vi "Controller Test Bench (9).vi"() -> ()   [LabVIEW 2022 SP3]
uses:
  <vilib>/sound2/lvsound2.llb/Sound Data Format.ctl
  <vilib>/Utility/error.llb/DialogType.ctl
  <vilib>/sound2/lvsound2.llb/Sampling Mode.ctl
  <vilib>/Analysis/4window.llb/windowTd.ctl
  <vilib>/DAQmx/read.llb/DAQmx Read (Analog 1D Wfm NChan NSamp).vi
  <vilib>/DAQmx/write.llb/DAQmx Write (Analog 1D DBL 1Chan NSamp).vi
  <vilib>/DAQmx/create/channels.llb/DAQmx Create Channel (AO-Voltage-Basic).vi
  <vilib>/DAQmx/create/channels.llb/DAQmx Create Channel (AI-Acceleration-Accelerometer).vi
  <vilib>/DAQmx/configure/timing.llb/DAQmx Timing (Sample Clock).vi
  <vilib>/DAQmx/miscellaneous.llb/DAQmx Fill In Error Info.vi
  <vilib>/DAQmx/configure/task.llb/DAQmx Configure Logging (TDMS).vi
  <vilib>/measure/maspectr.llb/FFT Spectrum (Mag-Phase) for N Chan.vi
  <vilib>/sound2/lvsound2.llb/Sound Output Set Volume (Single).vi
  <vilib>/sound2/lvsound2.llb/Sound Output Write (DBL Single).vi
  <vilib>/measure/NI_MAPro.lvlib
  <resource>/objmgr/daqmx.rc
  <vilib>/Analysis/NI_AALPro.lvlib
  <vilib>/measure/NI_MABase.lvlib
panel:
  in  "Gain":dbl
  in  "Setpoint":dbl
  out "Waveform Chart":waveform(dbl)[](graph)
  out "Numeric":i32
  in  "Output Noise":bool
  in  "reset signal":bool
  out "number of samples written per channel":u32
  in  "Active Control":bool
  in  "Log Data":bool
  out "Phase 2":cluster{"f0":dbl, "df":dbl, "phase":dbl[]}[](graph)
  out "Mag 2":cluster{"f0":dbl, "df":dbl, "magnitude":dbl[]}[](graph)
  in  "Show FFT":bool
  in  "Save FFT":bool
  in  "Start Acquisition":bool
  in  "Stop":bool
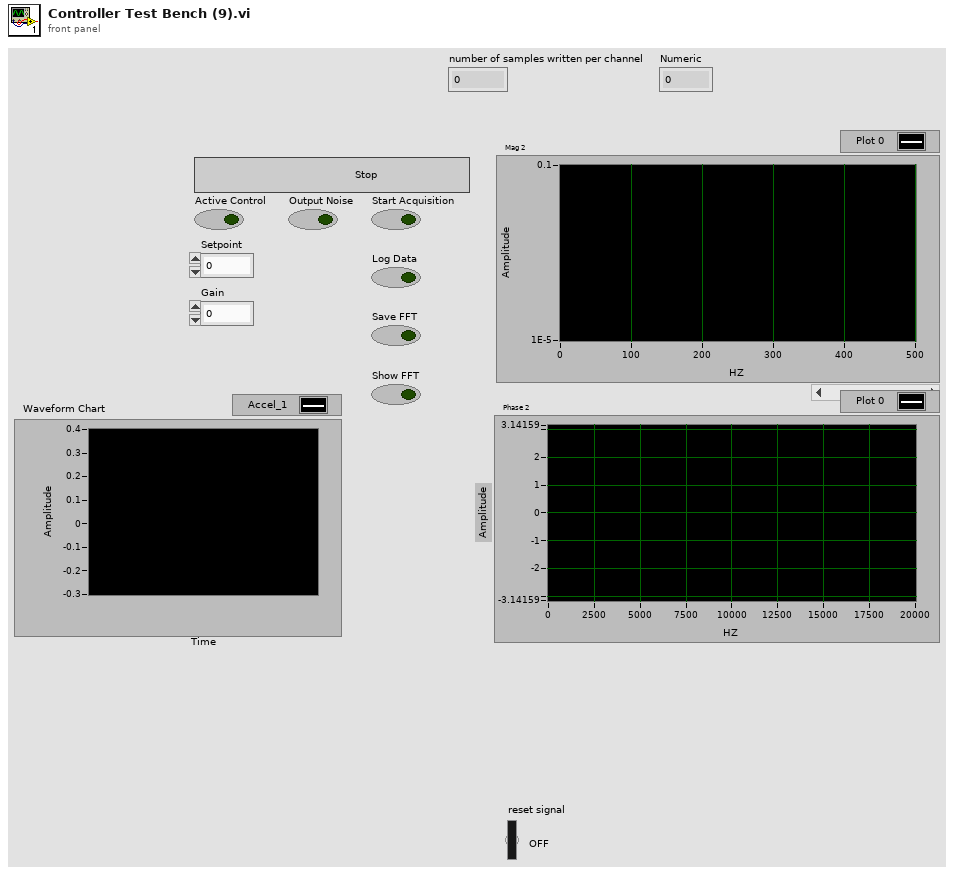
[diagram p1: front panel]
types:
  T1 = typedef "Sampling Mode.ctl" = i32
  T2 = typedef "DialogType.ctl" = u16
  T3 = typedef "Sound Data Format.ctl" = cluster{"sample rate (S/s)":dbl, "number of channels":i32, "bits per sample":i32}
  T4 = typedef "Sound Output Task ID.ctl" = u32
  T5 = typedef "NI_AALPro.lvlib/windowTd.ctl" = u32
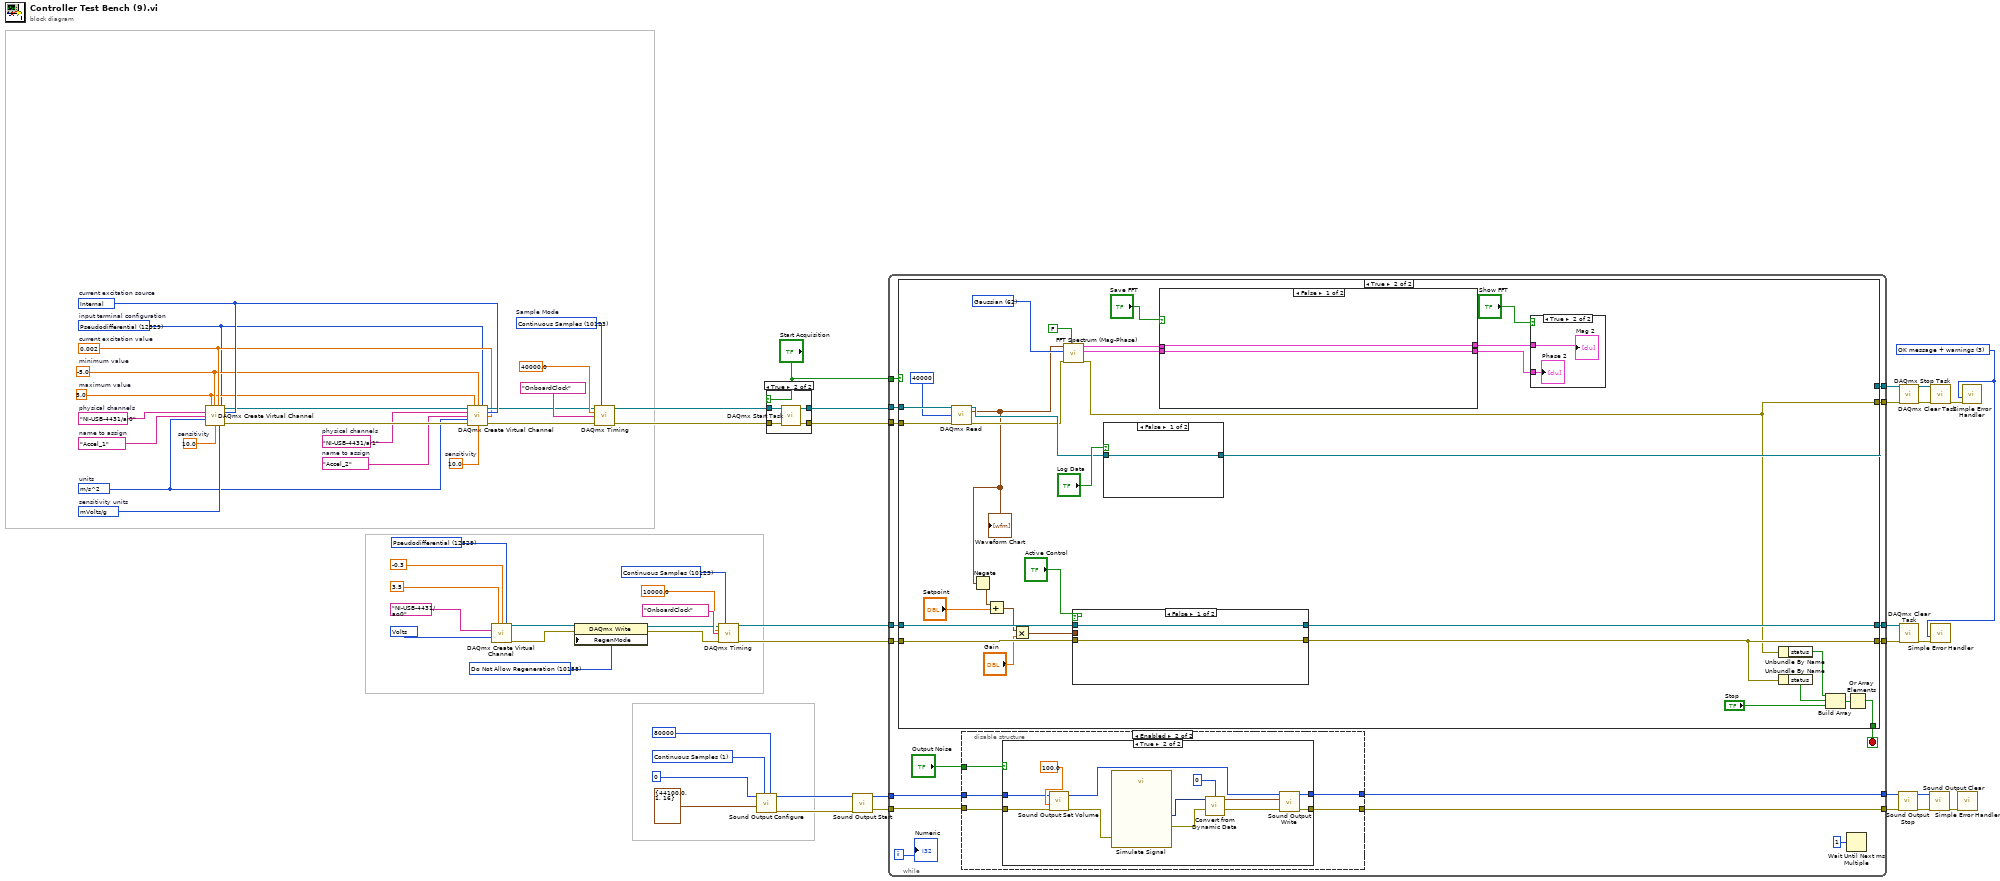
[diagram p0: block diagram]
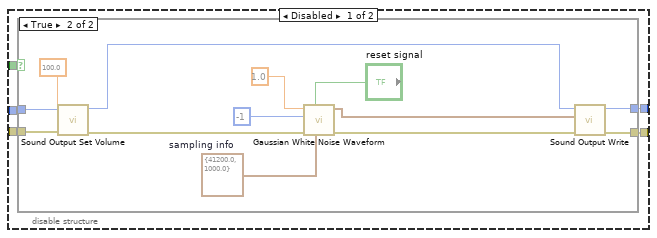
[diagram p3: hidden frame]
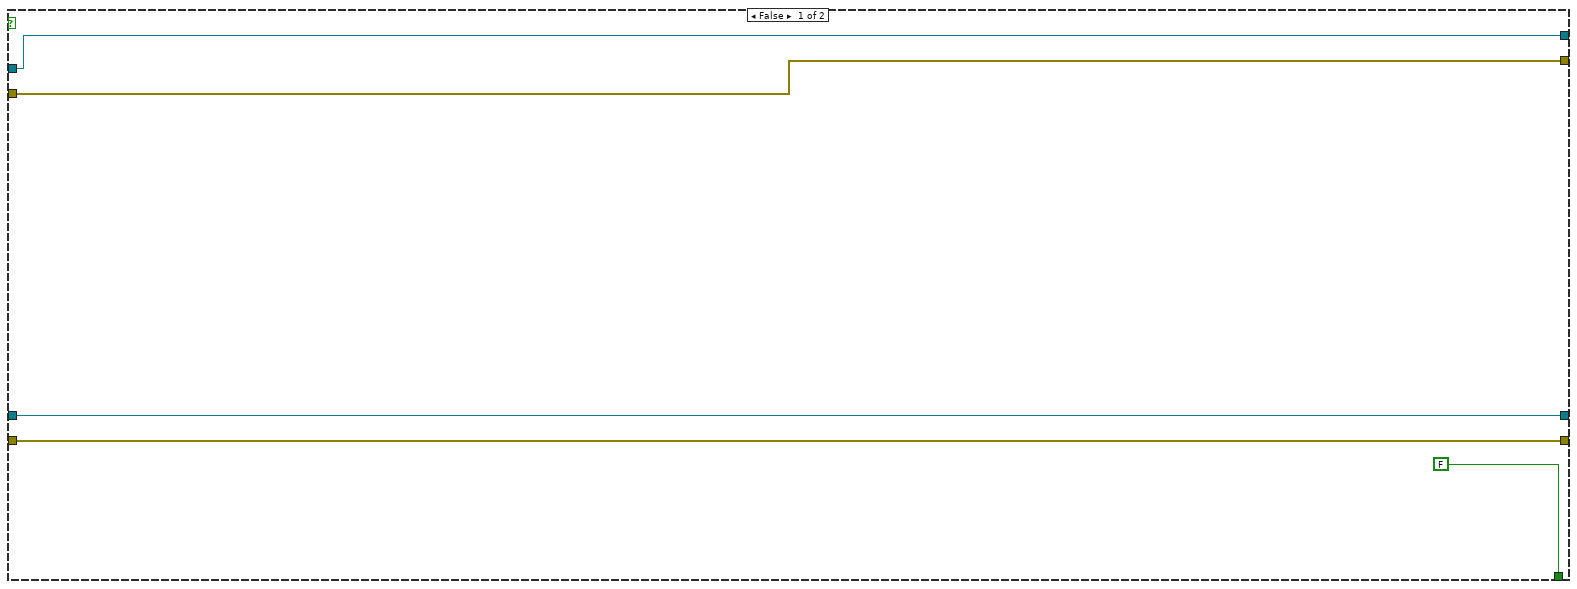
[diagram p6: hidden frame]
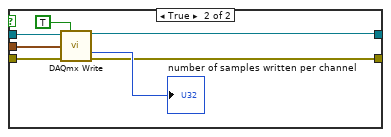
[diagram p7: hidden frame]
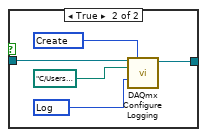
[diagram p10: hidden frame]
diagram:
  w3 = 10.0  # sensitivity
  w1 = tag "NI-USB-4431/ai1"  # physical channels
  w2 = "Accel_2"  # name to assign
  w28 = 10123 items=["Finite Samples"=10178, "Continuous Samples"=10123, "Hardware Timed Single Point"=12522] ("sample mode")
  w32 = 12509 items=["mVolts/g"=12509, "Volts/g"=12510]  # sensitivity units
  w33 = 10.0  # sensitivity
  w23 = 0.002  # current excitation value
  w26 = 10200 items=["Internal"=10200, "External"=10167, "None"=10230]  # current excitation source
  w17 = tag "NI-USB-4431/ai0"  # physical channels
  w31 = 10123 items=["Finite Samples"=10178, "Continuous Samples"=10123, "Hardware Timed Single Point"=12522]  # Sample Mode
  w19 = 12529 items=["default"=-1, "RSE"=10083, "NRSE"=10078, "Differential"=10106, "Pseudodifferential"=12529]  # input terminal configuration
  w22 = -5.0  # minimum value
  w21 = 5.0  # maximum value
  w34 = "Accel_1"  # name to assign
  w20 = 12470 items=["g"=10186, "m/s^2"=12470, "in/s^2"=12471, "From Custom Scale"=10065]  # units
  w35 = T1 1 items=["Finite Samples", "Continuous Samples"] ("sample mode")
  w46 = 10158 items=["Allow Regeneration"=10097, "Do Not Allow Regeneration"=10158] ("RegenMode")
  w36 = T2 3 items=["no dialog", "OK message", "continue or stop message", "OK message + warnings", "continue/stop + warnings"] ("type of dialog (OK msg:1)")
  w57 = 12529 items=["Default"=-1, "RSE"=10083, "Differential"=10106, "Pseudodifferential"=12529] ("output terminal configuration")
  w55 = 10348 items=["Volts"=10348, "From Custom Scale"=10065] ("units")
  n1 = call-poly <vilib>:"DAQmx Create Virtual Channel.vi"("maximum value"=w21, "minimum value"=w22, "input terminal configuration"=w19, "physical channels"=w17, "current excitation source"=w26, "name to assign"=w34, "current excitation value"=w23, "units"=w20, "sensitivity"=w33, "sensitivity units"=w32) -> ("task out"=w18:refnum<k21>, "error out"=w27:errorcluster)  [unwired: 4 in]
  n2 = call-poly <vilib>:"DAQmx Create Virtual Channel.vi"("task in"=w18, "maximum value"=w21, "minimum value"=w22, "input terminal configuration"=w19, "physical channels"=w1, "current excitation source"=w26, "name to assign"=w2, "current excitation value"=w23, "units"=w20, "error in"=w27, "sensitivity"=w3) -> ("task out"=w25:refnum<k21>, "error out"=w24:errorcluster)  [unwired: 3 in]
  n3 = call-poly <vilib>:"DAQmx Create Virtual Channel.vi"("maximum value"=3.5, "minimum value"=-0.3, "output terminal configuration"=w57, "physical channels"=tag "NI-USB-4431/ao0", "units"=w55) -> ("task out"=w43:refnum<k21>, "error out"=w47:errorcluster)  [unwired: 9 in]
  n4 = property class="DAQmx Write"(reference=w43, error in=w47, "RegenMode"=w46) -> (reference out=w41:refnum<k21>, error out=w42:errorcluster)
  n5 = call-poly <vilib>:"DAQmx Timing.vi"("task/channels in"=w25, "sample mode"=w31, "rate"=40000.0 ("Sample Rate"), "source"=tag "OnboardClock" ("Sample Clock Source"), "error in"=w24) -> ("task out"=w15:refnum<k21>, "error out"=w16:errorcluster)  [unwired: 9 in]
  n6 = call-poly <vilib>:"DAQmx Timing.vi"("task/channels in"=w41, "sample mode"=w28, "rate"=10000.0 ("Sample Rate"), "source"=tag "OnboardClock" ("Sample Clock Source"), "error in"=w42) -> ("task out"=w45:refnum<k21>, "error out"=w44:errorcluster)  [unwired: 9 in]
  n7 = call <vilib>:"Sound Output Configure.vi"("number of samples/ch"=80000 ("Number of Samples/ch"), "sample mode"=w35, "sound format"=T3 {"sample rate (S/s)"=44100.0, "number of channels"=1, "bits per sample"=16} ("Sound Format"), "device ID"=u32 0 ("Device ID")) -> ("error out"=w7:errorcluster, "task ID"=w6:T4)  [unwired: 6 in]
  n8 = case shown="True" "Start Acquisition" {
    tunnel: w16 -> [w63 w68]
    tunnel: w15 -> [w64 w67]
    tunnel: [w64 w66] -> w4
    tunnel: [w63 w65] -> w5
    frame False {
    }
    frame True {
      n9 = call <vilib>:"DAQmx Start Task.vi"("task/channels in"=w67, "error in"=w68) -> ("task out"=w66:refnum<k21>, "error out"=w65:errorcluster)  [unwired: 12 in]
    }
  }
  n10 = call <vilib>:"Sound Output Start.vi"("error in (no error)"=w7, "task ID"=w6) -> ("error out"=w8:errorcluster, "task ID out"=w9:T4)  [unwired: 8 in]
  n11 = while {
    tunnel: w8 -> [w74]
    tunnel: w9 -> [w75]
    tunnel: w4 -> [w84]
    tunnel: w5 -> [w69]
    tunnel: [w82] -> w51
    tunnel: [w83] -> w50
    tunnel: w45 -> [w81]
    tunnel: w44 -> [w80]
    tunnel: [w78] -> w40
    tunnel: [w79] -> w39
    tunnel: "Start Acquisition" -> [w77]
    tunnel: [w72] -> w11
    tunnel: [w71] -> w10
    tunnel: [w69] -> _
    i -> [w73]
    stop <- w85 stop-if-true
    n12 = case shown="True" w77 {
      tunnel: [FALSE w160] -> w85
      tunnel: w84 -> [w128 w159]
      tunnel: w69 -> [w127 w158]
      tunnel: [w128 w155] -> w83
      tunnel: [w127 w138] -> w82
      tunnel: w81 -> [w126 w145]
      tunnel: w80 -> [w125 w143]
      tunnel: [w126 w142] -> w79
      tunnel: [w125 w141] -> w78
      frame False {
      }
      frame True {
        w137 = T5 62 items=["Rectangle"=0, "Hanning"=1, "Hamming"=2, "Blackman-Harris"=3, "Exact Blackman"=4, "Blackman"=5, "Flat Top"=6, "4 Term B-Harris "=7, "7 Term B-Harris"=8, "Low Sidelobe"=9, "Blackman Nuttall"=11, "Triangle"=30, "Bartlett-Hanning"=31, "Bohman"=32, "Parzen"=33, "Welch"=34, "Kaiser"=60, "Dolph-Chebyshev"=61, "Gaussian"=62] ("window")
        n13 = call-poly <vilib>:"DAQmx Read.vi"("task/channels in"=w159, "number of samples per channel"=40000, "error in"=w158) -> ("task out"=w156:refnum<k21>, "data"=w132:waveform(dbl)[], "error out"=w139:errorcluster)  [unwired: 10 in]
        "Waveform Chart" <- w132
        n14 = Negate(x=w132) -> (-x=w130:waveform(dbl)[])
        n15 = Add(x=w130, y="Setpoint") -> (x+y=w129:waveform(dbl)[])
        n16 = Multiply(x=w129, y="Gain") -> (x*y=w144:waveform(dbl)[])
        n17 = call-poly <vilib>:"FFT Spectrum (Mag-Phase).vi"("restart averaging (F)"=FALSE, "error in (no error)"=w139, "window"=w137, "time signals"=w132) -> ("error out"=w138:errorcluster, "phases"=w149:cluster{"f0":dbl, "df":dbl, "phase":dbl[]}[], "magnitudes"=w150:cluster{"f0":dbl, "df":dbl, "magnitude":dbl[]}[])  [unwired: 3 in, 2 out]
        n18 = case shown="False" "Active Control" {
          tunnel: w143 -> [w162 w167]
          tunnel: [w161 w164] -> w142
          tunnel: [w162 w165] -> w141
          tunnel: w145 -> [w161 w169]
          tunnel: w144 -> [_ w168]
          frame False {
          }
          frame True {
            n19 = call-poly <vilib>:"DAQmx Write.vi"("task/channels in"=w169, "auto start"=TRUE, "data"=w168, "error in"=w167) -> ("task out"=w164:refnum<k21>, "number of samples written per channel"=→"number of samples written per channel":u32, "error out"=w165:errorcluster)  [unwired: 9 in]
          }
        }
        n20 = case shown="False" "Log Data" {
          tunnel: w156 -> [w176 w178]
          tunnel: [w176 w177] -> w155
          frame False {
          }
          frame True {
            w179 = 15848 items=["Open"=10437, "Open or Create"=15846, "Create or Replace"=15847, "Create"=15848] ("operation")
            w180 = 15844 items=["Off"=10231, "Log"=15844, "Log and Read"=15842] ("logging mode")
            n21 = call-poly <vilib>:"DAQmx Configure Logging.vi"("task/channels in"=w178, "operation"=w179, "file path"=path "C:/Users/LAV-UFSC/Documents/LAV - TCC", "logging mode"=w180) -> ("task out"=w177:refnum<k21>)  [unwired: 10 in, 1 out]
          }
        }
        n22 = case shown="False" "Save FFT" {
          tunnel: w150 -> [w170 w173]
          tunnel: w149 -> [w171 w172]
          tunnel: [w171 w172] -> w148
          tunnel: [w170 w173] -> w147
          frame False {
          }
          frame True {
          }
        }
        n23 = case shown="True" "Show FFT" {
          tunnel: w147 -> [_ w175]
          tunnel: w148 -> [_ w174]
          frame False {
          }
          frame True {
            "Mag 2" <- w175
            "Phase 2" <- w174
          }
        }
        n24 = Unbundle By Name(w138) -> ("status"=w135:bool)
        n25 = Unbundle By Name(w141) -> ("status"=w146:bool)
        n26 = Build Array(w135, w146, "Stop") -> (w153:bool[])
        n27 = Or Array Elements(Boolean array=w153) -> (logical OR=w160:bool)
      }
    }
    n28 = disable-structure shown="Enabled" {
      disable-tunnel: "Output Noise" -> [w90 w110]
      disable-tunnel: w75 -> [w89 w108]
      disable-tunnel: w74 -> [w88 w109]
      disable-tunnel: [w87 w107] -> w72
      disable-tunnel: [w86 w106] -> w71
      frame Disabled {
        n29 = case shown="True" w90 {
          tunnel: w88 -> [w91 w102]
          tunnel: w89 -> [w92 w103]
          tunnel: [w92 w105] -> w86
          tunnel: [w91 w104] -> w87
          frame False {
          }
          frame True {
            w93 = cluster{"Fs":dbl, "#s":dbl} {"Fs"=41200.0, "#s"=1000.0}  # sampling info
            n30 = call-poly <vilib>:"Sound Output Set Volume.vi"("error in (no error)"=w102, "volume"=100.0, "task ID"=w103) -> ("error out"=w99:errorcluster, "task ID out"=w101:T4)  [unwired: 7 in]
            n31 = call <vilib>:"Gaussian White Noise Waveform.vi"("sampling info"=w93, "reset signal"="reset signal", "error in (no error)"=w99, "seed"=-1, "standard deviation"=1.0) -> ("error out"=w98:errorcluster, "signal out"=w97:waveform(dbl))  [unwired: 5 in]
            n32 = call-poly <vilib>:"Sound Output Write.vi"("error in (no error)"=w98, "data"=w97, "task ID"=w101) -> ("error out"=w104:errorcluster, "task ID out"=w105:T4)  [unwired: 7 in]
          }
        }
      }
      frame Enabled {
        n33 = case shown="True" w110 {
          tunnel: w109 -> [w112 w116]
          tunnel: w108 -> [w111 w115]
          tunnel: [w112 w114] -> w107
          tunnel: [w111 w113] -> w106
          frame False {
          }
          frame True {
            n34 = call-poly <vilib>:"Sound Output Set Volume.vi"("error in (no error)"=w116, "volume"=100.0, "task ID"=w115) -> ("error out"=w121:errorcluster, "task ID out"=w120:T4)  [unwired: 7 in]
            n35 = call "Simulate Signal"("error in (no error)"=w121) -> ("DC with Gaussian Noise"=w123:dynamicdata, "error out"=w117:errorcluster)  [unwired: 13 in]
            n36 = call "Convert from Dynamic Data"("Dynamic Data Type"=w123, "Channel"=0) -> ("Waveform"=w122:waveform(dbl))  [unwired: 2 in]
            n37 = call-poly <vilib>:"Sound Output Write.vi"("error in (no error)"=w117, "data"=w122, "task ID"=w120) -> ("error out"=w114:errorcluster, "task ID out"=w113:T4)  [unwired: 7 in]
          }
        }
      }
    }
    n38 = Wait Until Next ms Multiple(millisecond multiple=u32 1) -> ()  [unwired: 1 out]
    "Numeric" <- w73
  }
  n39 = call <vilib>:"Sound Output Stop.vi"("error in (no error)"=w11, "task ID"=w10) -> ("error out"=w14:errorcluster, "task ID out"=w13:T4)  [unwired: 8 in]
  n40 = call <vilib>:"DAQmx Stop Task.vi"("task/channels in"=w50, "error in"=w51) -> ("task out"=w53:refnum<k21>, "error out"=w52:errorcluster)  [unwired: 12 in]
  n41 = call <vilib>:"DAQmx Clear Task.vi"("task in"=w39, "error in"=w40) -> ("error out"=w38:errorcluster)  [unwired: 13 in]
  n42 = call <vilib>:"Sound Output Clear.vi"("error in (no error)"=w14, "task ID"=w13) -> ("error out"=w12:errorcluster)  [unwired: 9 in]
  n43 = call <vilib>:"DAQmx Clear Task.vi"("task in"=w53, "error in"=w52) -> ("error out"=w54:errorcluster)  [unwired: 13 in]
  n44 = call <vilib>:"Simple Error Handler.vi"("type of dialog (OK msg:1)"=w36, "error in (no error)"=w38) -> ()  [unwired: 3 in, 5 out]
  n45 = call <vilib>:"Simple Error Handler.vi"("error in (no error)"=w12) -> ()  [unwired: 4 in, 5 out]
  n46 = call <vilib>:"Simple Error Handler.vi"("type of dialog (OK msg:1)"=w36, "error in (no error)"=w54) -> ()  [unwired: 3 in, 5 out]
